vi "FixUpVerasonicsEyeFiles.vi"() -> ()   [LabVIEW 2022 SP3]
panel:
  in  "Use Selected Files":bool
  in  "Listbox":i32[](listbox)
  in  "A/D info.# rf points per line":u16
  out "Syth Aperture 2":sgl[][](graph)
  out "Syth Aperture":sgl[][](graph)
  in  "directory path":path
  in  "pattern":string="*.eye"
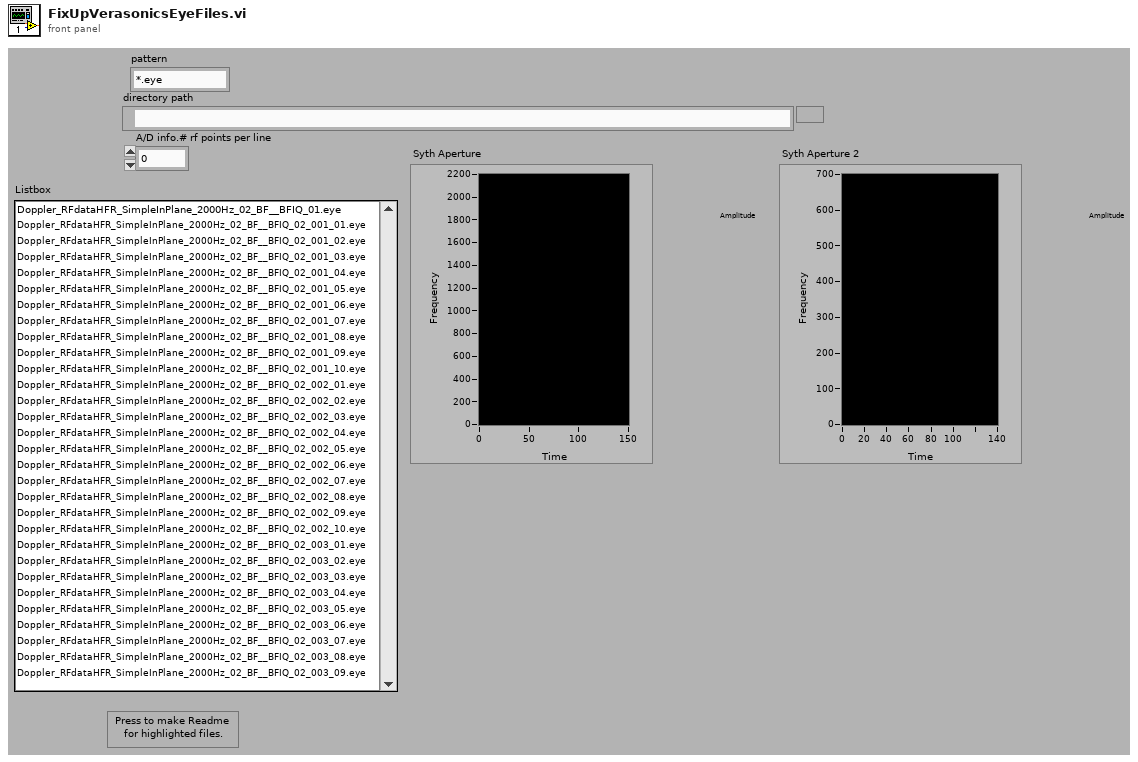
[diagram p1: front panel]
types:
  T1 = enum16{"big-endian, network order", "native, host order", "little-endian"}
  T2 = typedef "Header.ctl" = cluster{"header info":cluster{"Header":string, "Head length":i16}, "A/D info":cluster{"# rf points per line":u16, "# lines per scan":u16, "sample rate MHz":u16, "# A/D bits":i16, "# bytes per A/D":u16, "TGC Flag":u16, "A/D Type":string}, "Tranducer Info":cluster{"bandwidth":sgl, "center freq":sgl, "start freq":sgl, "ID":i32}, "Scan Info":cluster{"delay":sgl, "pivot distance":sgl, "sector scan angle":sgl, "operator":string, "Scan Mode":string, "location":string}, "Time/Date Info":cluster{"date":string, "time":string}, "RF Info":cluster{"RF file name":string, "RF file att":string, "RF cal file name":string, "RF cal file att":string}, "Patient Info":cluster{"ID":string, "extended ID":string, "age":u16, "sex":string, "previously\nscanned":string, "PSA":sgl, "LOS":u8, "Ethnicty 2":u8, "Race":u8}, "Tissue Type":cluster{"organ":i16, "disease type":i16, "disease location":i16, "IQ_pts":u16, "RcvBuffer":u8, "RcvFrame":u16, "IQBuff":u8, "IQFrame":u16, "IQPage":u8}, "Votage scaling":cluster{"Digitizer (dB)":sgl, "Gain (dB)":sgl, "Atten (dB)":sgl}, "Comment":string, "Misc Info":cluster{"avg num":u16, "c speed":i16, "Div By or SF zones":i16, "XMIT CHS":u8, "RCV CHS":u8, "Xmit angle":sgl}, "Therapy Parameters":cluster{"Theraputic Freq (MHz)":sgl, "Time on (s)":sgl, "Therapy amplitude (mV)":sgl, "Lines Before":u16, "Lines After":u16}, "Scan Settings":cluster{"Energy (uJ or V)":u8, "Damp (Ohm) or Fc":u8, "HP Filt (KHz)":u8, "LP Filt (MHz)":u8, "Gain (db)":u8, "prf (kHz)":sgl, "Distance between\nscan lines (um)":u16, "Distance between\nscan planes (um)":u16, "Scan line gap (um)":sgl, "Scan plane gap (um)":sgl}, "Compression Parameters":cluster{"F1 (MHz)":sgl, "F2 (MHz)":sgl, "% taper":sgl, "duration":sgl}, "Patient Info Xtra":cluster{"First Name":string, "Last Name":string, "Notes":string}, "ROI Box":u16[]}
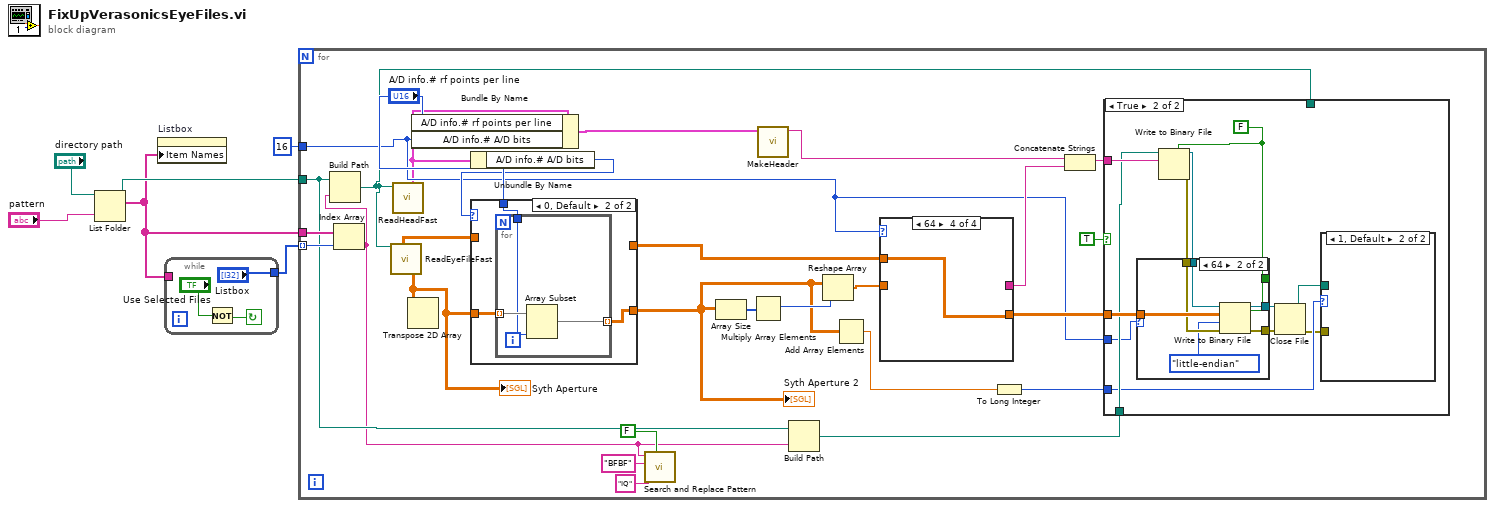
[diagram p0: block diagram]
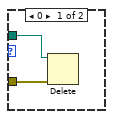
[diagram p3: hidden frame]
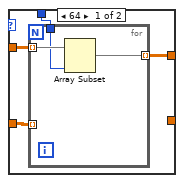
[diagram p5: hidden frame]
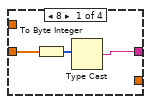
[diagram p6: hidden frame]
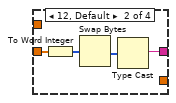
[diagram p7: hidden frame]
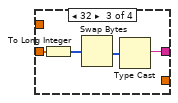
[diagram p8: hidden frame]
diagram:
  n1 = List Folder(path="directory path", pattern="pattern") -> (path out=w4:path, filenames=w2:string[])  [unwired: 1 in, 3 out]
  n2 = property on="Listbox" class="LstBox (strict)"("Item Names"=w2) -> ()  [unwired: 2 in, 2 out]
  n3 = while {
    tunnel: ["Listbox"] -> w3
    tunnel: w2 -> [_]
    stop <- w9 continue-if-true
    n4 = Not(x="Use Selected Files") -> (.not. x?=w9:bool)
  }
  n5 = for {
    tunnel: w4 -> [w21]
    tunnel: w3 -> [w27] mode=indexing
    tunnel: w2 -> [w26]
    tunnel: i16 16 ("A/D info.# A/D bits") -> [w14]
    n6 = Index Array(array=w26, index=w27) -> (element=w18:string)
    n7 = Build Path(base path=w21, name or relative path=w18) -> (appended path=w19:path)
    n8 = call "ReadEyeFileFast.vi"("new file path"=w19) -> ("Complex output array"=w32:csg[][], "2-D data array"=w15:sgl[][])  [unwired: 13 in, 4 out]
    "Syth Aperture" <- w15
    n9 = call "ReadHeadFast.vi"("new file path"=w19) -> ("Header In"=w10:T2)  [unwired: 7 in, 3 out]
    n10 = Transpose 2D Array(2D array=w15) -> ()  [unwired: 1 out]
    n11 = Bundle By Name(cluster=w10, "A/D info.# rf points per line"="A/D info.# rf points per line", "A/D info.# A/D bits"=w14) -> (w33:T2)
    n12 = Unbundle By Name(w10) -> ("A/D info.# A/D bits"=w17:i16)
    n13 = case shown="0, Default" w17 {
      tunnel: w32 -> [w64 _]
      tunnel: "A/D info.# rf points per line" -> [w63 w70]
      tunnel: [_ w68] -> w13
      tunnel: [w62 _] -> w30
      tunnel: w15 -> [w61 w69]
      frame 64 {
        n14 = for {
          tunnel: w61 -> [_] mode=indexing
          tunnel: w64 -> [w67] mode=indexing
          tunnel: [w66] -> w62 mode=indexing
          tunnel: w63 -> [w65]
          n15 = Array Subset(array=w67, length=w65) -> (w66:csg[])  [unwired: 1 in]
        }
      }
      frame 0, Default {
        n16 = for {
          tunnel: w69 -> [w73] mode=indexing
          tunnel: [w72] -> w68 mode=indexing
          tunnel: w70 -> [w71]
          n17 = Array Subset(array=w73, length=w71) -> (w72:sgl[])  [unwired: 1 in]
        }
      }
    }
    "Syth Aperture 2" <- w13
    n18 = call <vilib>:"Search and Replace Pattern.vi"("string"=w18, "regular expression (\"\")"="BFBF" ("substring (\"\")"), "replace string (\"\")"="IQ" ("replace string (\"\")"), "replace all? (F)"=FALSE) -> ()  [unwired: 1 in, 2 out]
    n19 = Array Size(array=w13) -> (size(s)=w36:i32[])
    n20 = Multiply Array Elements(1:w36) -> (0:w35:i32)
    n21 = call "MakeHeader.vi"("Header In"=w33) -> ("Header String"=w25:string)  [unwired: 6 in]
    n22 = Build Path(base path=w21, name or relative path=w18) -> (appended path=w22:path)
    n23 = Reshape Array(w13, w35) -> (w37:sgl[])
    n24 = Add Array Elements(numeric array=w13) -> (sum=w12:sgl)
    n25 = case shown="64" w14 {
      tunnel: w37 -> [w75 w80 w84 _]
      tunnel: [w76 w79 w83 _] -> w34
      tunnel: w30 -> [_ _ _ w85]
      tunnel: [_ _ _ w85] -> w29
      frame 8 {
        n26 = To Byte Integer(number=w75) -> (8bit integer=w74:i8[])
        n27 = Type Cast(x=w74) -> (*(type *) &x=w76:string)  [unwired: 1 out]
      }
      frame 12, Default {
        n28 = To Word Integer(number=w80) -> (16bit integer=w77:i16[])
        n29 = Swap Bytes(anything=w77) -> (byte swapped=w78:i16[])
        n30 = Type Cast(x=w78) -> (*(type *) &x=w79:string)  [unwired: 1 out]
      }
      frame 32 {
        n31 = To Long Integer(number=w84) -> (32bit integer=w81:i32[])
        n32 = Swap Bytes(anything=w81) -> (byte swapped=w82:i32[])
        n33 = Type Cast(x=w82) -> (*(type *) &x=w83:string)  [unwired: 1 out]
      }
      frame 64 {
      }
    }
    n34 = To Long Integer(number=w12) -> (32bit integer=w11:i32)
    n35 = Concatenate Strings(w25, w34) -> (w28:string)
    n36 = case shown="True" TRUE {
      tunnel: w29 -> [_ w49]
      tunnel: w28 -> [_ w48]
      tunnel: w22 -> [_ w42]
      tunnel: w19 -> [_ _]
      tunnel: w14 -> [_ w41]
      tunnel: w11 -> [_ w40]
      frame False {
      }
      frame True {
        w47 = FALSE ("prepend array or string size? (T)")
        n37 = Write to Binary File(file (use dialog)=w42, data=w48, 5:w47) -> (refnum out=w46:refnum<file>, error out=w45:errorcluster)  [unwired: 3 in, 1 out]
        n38 = case shown="64" w41 {
          tunnel: w49 -> [_ w60]
          tunnel: w47 -> [_ w59]
          tunnel: w46 -> [w53 w58]
          tunnel: w45 -> [w52 w57]
          tunnel: [w52 w56] -> w44
          tunnel: [w53 w55] -> w43
          frame 0, Default {
          }
          frame 64 {
            n39 = Write to Binary File(file (use dialog)=w58, data=w60, error in=w57, 5:w59, 9:T1."little-endian" ("byte order (0:big-endian, network order)")) -> (refnum out=w55:refnum<file>, error out=w56:errorcluster)  [unwired: 1 in, 1 out]
          }
        }
        n40 = Close File(refnum=w43, error in=w44) -> (path=w39:path, error out=w38:errorcluster)
        n41 = case shown="1, Default" w40 {
          tunnel: w39 -> [w51 _]
          tunnel: w38 -> [w50 _]
          frame 0 {
            n42 = Delete(path (use dialog)=w51, error in=w50) -> ()  [unwired: 3 in, 3 out]
          }
          frame 1, Default {
          }
        }
      }
    }
  }
